vi "Symphony Datasocket test.vi"() -> ()   [LabVIEW 2012]
panel:
  in  "stop":bool
  out "timed out":bool
  out "data":cluster{"Message":string, "Data":variant, i32}
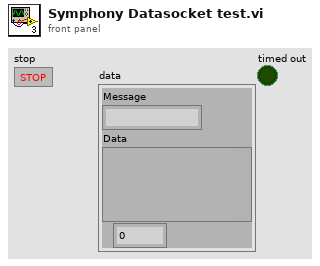
[diagram p1: front panel]
types:
  T1 = enum16{"Read", "Write", "ReadWrite", "BufferedRead", "BufferedReadWrite"}
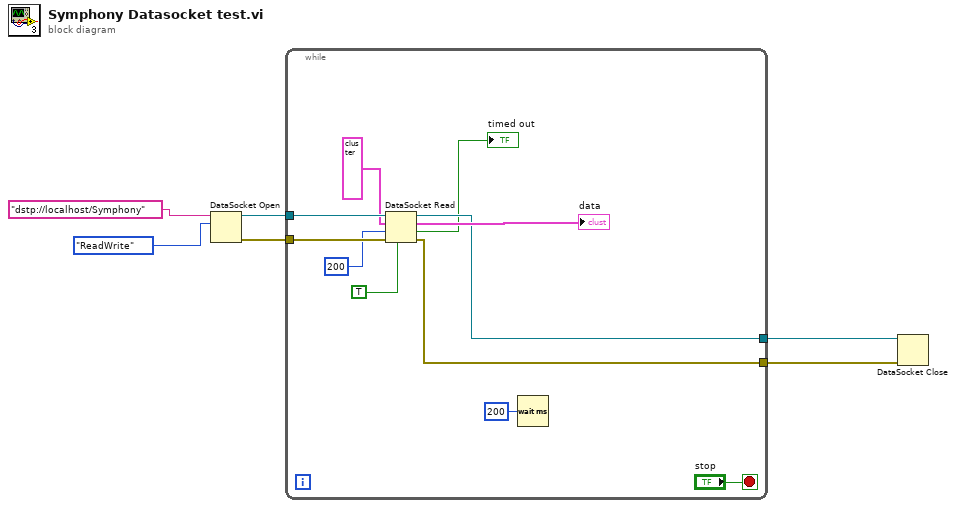
[diagram p0: block diagram]
diagram:
  n1 = DataSocket Open(10:T1."ReadWrite" ("mode"), 11:"dstp://localhost/Symphony" ("URL")) -> (0:w5:errorcluster, 3:w6:refnum<k13>)  [unwired: 2 in]
  n2 = while {
    tunnel: w6 -> [w17]
    tunnel: w5 -> [w16]
    tunnel: [w13] -> w4
    tunnel: [w12] -> w3
    stop <- "stop" stop-if-true
    n3 = DataSocket Read(6:TRUE ("wait for updated value (T)"), 8:w16, 9:200 ("ms timeout (10000)"), 10:cluster{"Message":string, "Data":variant, i32} {"Message"="", "Data"=variant, 0} ("SympClient"), 11:w17) -> (0:w12:errorcluster, 1:→"timed out":bool, 2:→"data":cluster{"Message":string, "Data":variant, i32}, 3:w13:refnum<k13>)  [unwired: 3 out]
    n4 = Wait (ms)(milliseconds to wait=u32 200) -> ()  [unwired: 1 out]
  }
  n5 = DataSocket Close(8:w3, 11:w4) -> ()  [unwired: 1 in, 2 out]
